vi "xy_preprocessing.vi"(9 "XY correction":bool, 10 "approach":bool, 11 "all rows":dbl[][](array[numeric])) -> (2 "Numeric":dbl, 3 "Numeric 2":dbl)   [LabVIEW 2015]
uses:
  <vilib>/Analysis/NI_AALBase.lvlib
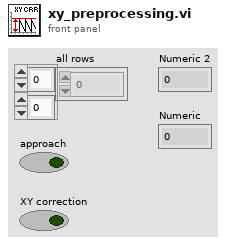
[diagram p1: front panel]
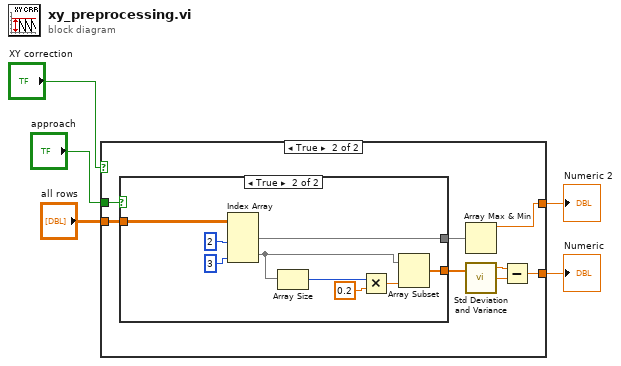
[diagram p0: block diagram]
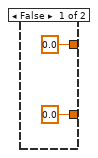
[diagram p2: hidden frame]
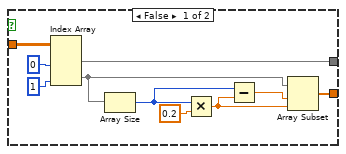
[diagram p3: hidden frame]
diagram:
  n1 = case shown="True" "XY correction" {
    tunnel: [0.0 w15] -> w1
    tunnel: [0.0 w12] -> w2
    tunnel: "approach" -> [_ w11]
    tunnel: "all rows" -> [_ w10]
    frame False {
    }
    frame True {
      n2 = case shown="True" w11 {
        tunnel: w10 -> [w18 w28]
        tunnel: [w19 w27] -> w9
        tunnel: [w17 w26] -> w8
        frame False {
          n3 = Index Array(array=w18, index (col) #1=0 ("disabled index (col)"), index (col) #2=1 ("index (col)")) -> (element #1=w17:dbl[], element #2=w24:dbl[])  [unwired: 2 in]
          n4 = Array Size(array=w24) -> (size(s)=w25:i32)
          n5 = Multiply(x=w25, y=0.2) -> (x*y=w16:dbl)
          n6 = Subtract(x=w25, y=w16) -> (x-y=w20:dbl)
          n7 = Array Subset(array=w24, index=w20, length=w16) -> (w19:dbl[])
        }
        frame True {
          n8 = Index Array(array=w28, index (col) #1=2 ("disabled index (col)"), index (col) #2=3 ("index (col)")) -> (element #1=w26:dbl[], element #2=w32:dbl[])  [unwired: 2 in]
          n9 = Array Size(array=w32) -> (size(s)=w34:i32)
          n10 = Multiply(x=w34, y=0.2) -> (x*y=w33:dbl)
          n11 = Array Subset(array=w32, length=w33) -> (w27:dbl[])  [unwired: 1 in]
        }
      }
      n12 = Array Max & Min(array=w8) -> (max value=w15:dbl)  [unwired: 3 out]
      n13 = call <vilib>:"Std Deviation and Variance.vi"("X"=w9) -> ("mean"=w14:dbl, "standard deviation"=w13:dbl)  [unwired: 1 in, 1 out]
      n14 = Subtract(x=w14, y=w13) -> (x-y=w12:dbl)
    }
  }
  "Numeric" <- w2
  "Numeric 2" <- w1
